vi "Multiple Connections Server Template.vi"() -> ()   [LabVIEW 2013, in "Connection_GOSPL.lvlib" / "Connection.Collection.lvclass"]
uses:
  Connection.Collection.lvclass
  Connection/Connection.lvclass
  Connection.TCP/Connection.TCP.lvclass
  Connection.LocalQueue/Connection.LocalQueue.lvclass
panel:
  out "listener error":errorcluster
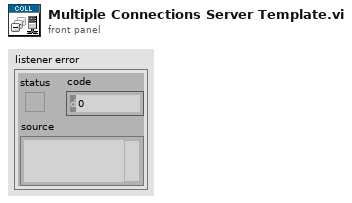
[diagram p1: front panel]
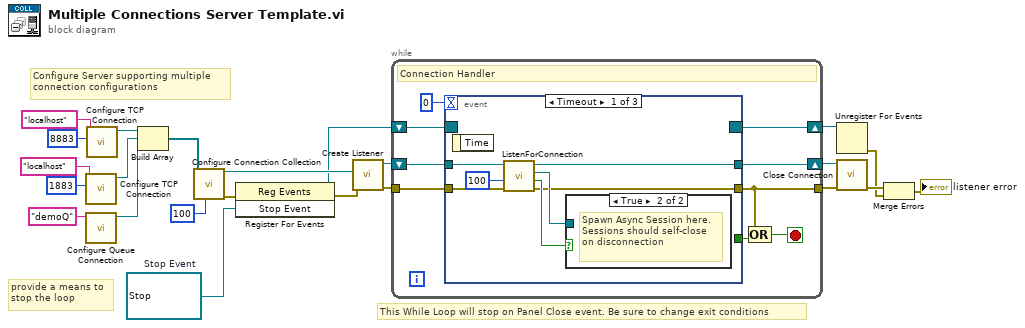
[diagram p0: block diagram]
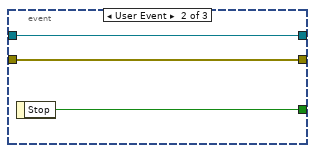
[diagram p3: hidden frame]
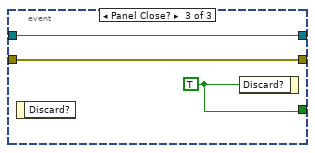
[diagram p4: hidden frame]
diagram:
  w11 = refnum<user-event> refnum  # Stop Event
  # "This While Loop will stop on Panel Close event. Be sure to change exit conditions"
  # "provide a means to\nstop the loop"
  # "Configure Server supporting multiple\nconnection configurations"
  n1 = call "Configure TCP Connection.vi"("remote port (80)"=u16 1883, "address (localhost)"="localhost") -> ("Connection.TCP"=w4:refnum<class "Connection.TCP.lvclass">)  [unwired: 8 in, 1 out]
  n2 = call "Configure Queue Connection.vi"("Queue Name"="demoQ") -> ("Connection.LocalQueue"=w2:refnum<class "Connection.LocalQueue.lvclass">)  [unwired: 9 in, 1 out]
  n3 = call "Configure TCP Connection.vi"("remote port (80)"=u16 8883, "address (localhost)"="localhost") -> ("Connection.TCP"=w7:refnum<class "Connection.TCP.lvclass">)  [unwired: 8 in, 1 out]
  n4 = Build Array(w7, w4, w2) -> (w1:refnum<class "Connection.lvclass">[])
  n5 = call "Configure Connection Collection.vi"("timeout (-1: Connection Default)"=100, "Collection"=w1) -> ("error out"=w14:errorcluster, "Connection"=w23:refnum<class "Connection.Collection.lvclass">)  [unwired: 8 in]
  n6 = register-events(error in=w14, w11) -> (reference out=w13:refnum<event-registration>, error out=w12:errorcluster)  [unwired: 1 in]
  n7 = call "Create Listener.vi"("error in (no error)"=w12, "Connection Configuration"=w23) -> ("error out"=w21:errorcluster, "Listener"=w22:refnum<class "Connection.lvclass">)  [unwired: 8 in]
  n8 = while {
    tunnel: w21 -> [w31]
    tunnel: [w29] -> w19
    shift-right: [w30] -> w20
    shift-left: w22 -> [w32]
    shift-right: [w26] -> w18
    shift-left: w13 -> [w25]
    stop <- w28 stop-if-true
    # "Connection Handler"
    n9 = event shown="[0] Timeout" {
      selector: w25 -> [_ _ _]
      dyn-events: [_ _ _] -> w26
      timeout: 0 -> [_ _ _]
      tunnel: w32 -> [w38 w42 w45]
      tunnel: w31 -> [w35 w41 w44]
      tunnel: [w34 w42 w45] -> w30
      tunnel: [w33 w41 w44] -> w29
      tunnel: [_ w40 w43] -> w24
      event Timeout {
        n10 = event-data() -> ()  [unwired: 1 in, 1 out]
        n11 = call "ListenForConnection.vi"("error in (no error)"=w35, "timeout (2000 ms)"=100 ("bytes to read (100)"), "Listener"=w38) -> ("error out"=w33:errorcluster, "New connection"=w36:bool, "Connection"=w37:refnum<class "Connection.lvclass">, "Listener out"=w34:refnum<class "Connection.lvclass">)  [unwired: 5 in]
        n12 = case shown="True" w36 {
          tunnel: w37 -> [_ _]
          frame False {
          }
          frame True {
            # "Spawn Async Session here. Sessions should self-close on disconnection"
          }
        }
      }
      event User Event {
        n13 = event-data() -> ("Stop"=w40:bool)  [unwired: 1 in]
      }
      event Panel Close? {
        w43 = TRUE ("Discard?")
        n14 = event-data() -> ()  [unwired: 1 in, 1 out]
        n15 = event-data("Discard?"=w43) -> ()  [unwired: 1 in, 1 out]
      }
    }
    n16 = Compound Arithmetic op=OR(w29, w24) -> (w28:bool)
  }
  n17 = Unregister For Events(event registration refnum=w18) -> (error out=w15:errorcluster)  [unwired: 1 in]
  n18 = call "Close Connection.vi"("error in (no error)"=w19, "Connection in"=w20) -> ("error out"=w17:errorcluster)  [unwired: 8 in, 1 out]
  n19 = Merge Errors(w17, w15) -> (→"listener error":errorcluster)
